vi "Validate Command.vi"(4 "error in (no error)":errorcluster, 7 "Serial in":refnum<visa-resource-name>) -> (0 "error out":errorcluster, 2 "Valid?":bool, 3 "Serial Out":refnum<visa-resource-name>)   [LabVIEW 2019, in "Faulhaber RS232.lvlib"]
uses:
  Faulhaber RS232.lvlib
  <vilib>/Utility/error.llb/Error Cluster From Error Code.vi
  <vilib>/ErrorRing/Error Ring.xnode
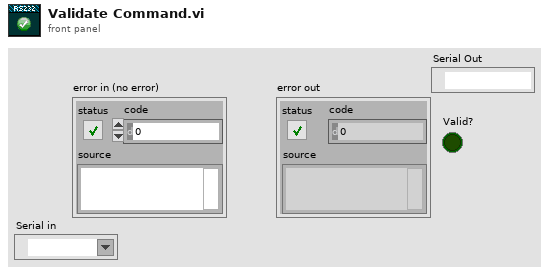
[diagram p1: front panel]
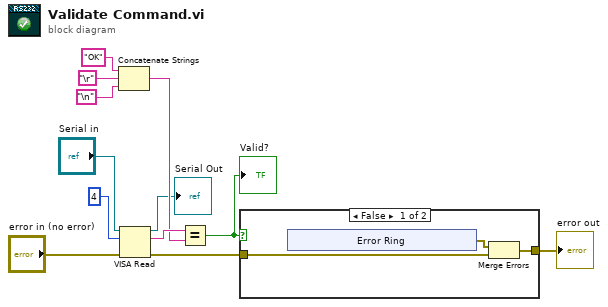
[diagram p0: block diagram]
diagram:
  n1 = Concatenate Strings("OK" ("y"), "\r", "\n") -> (w8:string)
  n2 = VISA Read(VISA resource name="Serial in", byte count=u32 4, error in (no error)="error in (no error)") -> (VISA resource name out=→"Serial Out":refnum<visa-resource-name>, read buffer=w9:string, error out=w4:errorcluster)  [unwired: 1 out]
  n3 = Equal?(x=w9, y=w8) -> (x = y?=w10:bool)
  "Valid?" <- w10
  n4 = case shown="False" w10 {
    tunnel: [w15 w21] -> w11
    tunnel: w4 -> [w13 w21]
    frame False {
      n5 = xnode "Error Ring"() -> ("error out"=w14:errorcluster)
      n6 = Merge Errors(w14, w13) -> (w15:errorcluster)
    }
    frame True {
    }
  }
  "error out" <- w11
